vi "FTW-Subscriber-Destroy.vi"(0 "FTW-Subscription In":refnum<class "FTW-Subscriber.lvclass">, 11 "error in":errorcluster) -> (15 "error out":errorcluster)   [LabVIEW 2013, in "FTW-Subscriber.lvclass"]
uses:
  FTW-Subscriber.lvclass
  FTW-Subscriber.lvclass/FTW-Subscriber.ctl
  Package/Lossy/FTW-Package-Lossy.lvclass
  Endpoint/FTW-Endpoint.lvclass
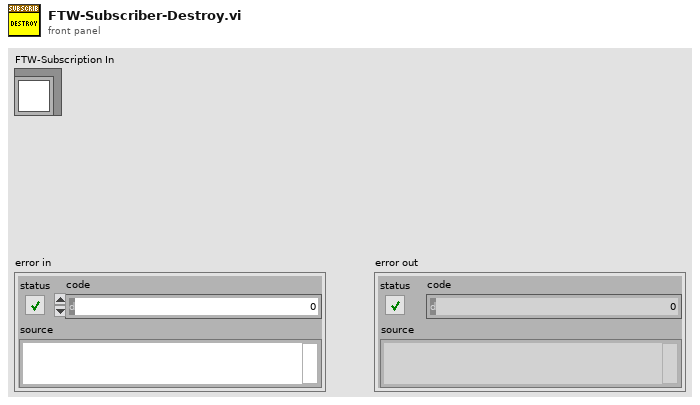
[diagram p1: front panel]
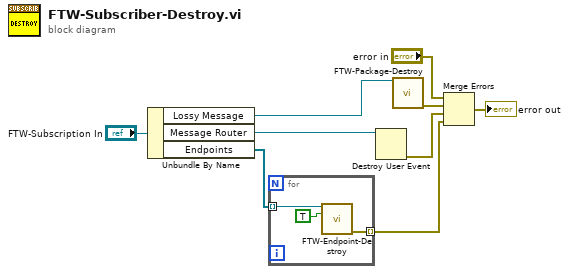
[diagram p0: block diagram]
diagram:
  n1 = Unbundle By Name("FTW-Subscription In") -> ("Lossy Message"=w2:refnum<class "FTW-Package-Lossy.lvclass">, "Message Router"=w6:refnum<user-event>, "Endpoints"=w4:refnum<class "FTW-Endpoint.lvclass">[])
  n2 = for {
    tunnel: w4 -> [w12] mode=indexing
    tunnel: [w11] -> w3 mode=indexing
    n3 = call-dynamic "FTW-Endpoint-Destroy.vi"("FTW Endpoint"=w12, "Force Destroy"=TRUE ("force destroy? (F)")) -> ("error out"=w11:errorcluster)  [unwired: 13 in]
  }
  n4 = Destroy User Event(user event=w6) -> (error out=w5:errorcluster)  [unwired: 1 in]
  n5 = call-dynamic "FTW-Package-Destroy.vi"("FTW Lossy Message"=w2) -> ("error out"=w1:errorcluster)  [unwired: 14 in]
  n6 = Merge Errors("error in", w1, w5, w3) -> (→"error out":errorcluster)
